vi "get image.vi"(8 "error in (no error)":errorcluster, 11 "Camera Process in":refnum<class "Camera Process.lvclass">) -> (0 "error out":errorcluster, 3 "Camera Process out":refnum<class "Camera Process.lvclass">)   [LabVIEW 2022 SP3, in "Cam Process.lvlib" / "Camera Process.lvclass"]
uses:
  Camera Process.lvclass
  Camera Process.lvclass/Camera Process.ctl
  Camera Driver/Camera Driver.lvclass
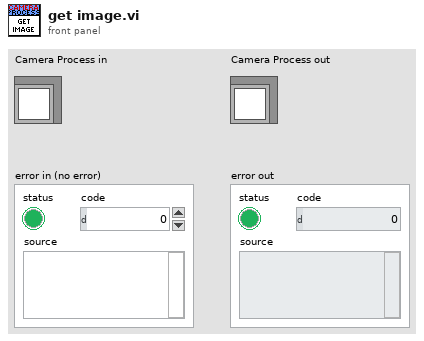
[diagram p1: front panel]
types:
  T1 = typedef "IMAQ Image.ctl" = refnum<image>
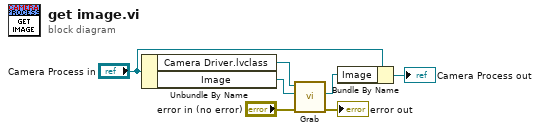
[diagram p0: block diagram]
diagram:
  n1 = Unbundle By Name("Camera Process in") -> ("Camera Driver.lvclass"=w2:refnum<class "Camera Driver.lvclass">, "Image"=w1:T1)
  n2 = call-dynamic "Grab.vi"("error in (no error)"="error in (no error)", "Image"=w1, "Camera Driver in"=w2) -> ("error out"=→"error out":errorcluster, "Image out"=w4:T1)  [unwired: 6 in, 1 out]
  n3 = Bundle By Name(cluster="Camera Process in", "Image"=w4) -> (→"Camera Process out":refnum<class "Camera Process.lvclass">)
